vi "McP Position Limit Checker.vi"(1 "Scanning Step":dbl=100.0 min=0.0 format="%.4f", 2 "Old Counter Position":dbl=619.92122 min=0.0 format="%.4f", 3 "New Counter Position":dbl=619.92122 min=0.0 format="%.4f") -> (0 "New Counter Position output":dbl=619.92122 format="%.4f")   [LabVIEW 2025]
doc: "Author: Scott Hannahs <sth@magnet.fsu.edu>\n\nThis software is licensed for use under the “MIT License\"\nCopyright (c) 2025 Scott Hannahs, sth@sth@magnet.sthnet.net\n\nPermission is hereby granted, free of charge, to any person obtaining a copy of this software and associated documentation files (the \"Software\"), to deal in the Software without restriction, including without limitation the rights to use, copy, modify, merge, publish, distribute, sublicense, and/or sell copies of the Software, and to permit persons to whom the Software is furnished to do so, subject to the following conditions: The above copyright notice and this permission notice shall be included in all copies or substantial portions of the Software.\n\nTHE SOFTWARE IS PROVIDED \"AS IS\", WITHOUT WARRANTY OF ANY KIND, EXPRESS OR IMPLIED, INCLUDING BUT NOT LIMITED TO THE WARRANTIES OF MERCHANTABILITY, FITNESS FOR A PARTICULAR PURPOSE AND NONINFRINGEMENT. IN NO EVENT SHALL THE AUTHORS OR COPYRIGHT HOLDERS BE LIABLE FOR ANY CLAIM, DAMAGES OR OTHER LIABILITY, WHETHER IN AN ACTION OF CONTRACT, TORT OR OTHERWISE, ARISING FROM, OUT OF OR IN CONNECTION WITH THE SOFTWARE OR THE USE OR OTHER DEALINGS IN THE SOFTWARE."
panel:
  out "Message":string
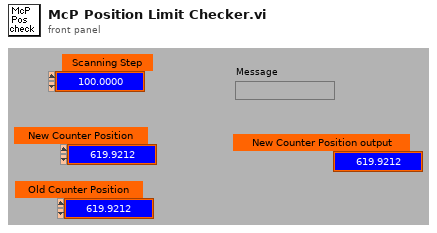
[diagram p1: front panel]
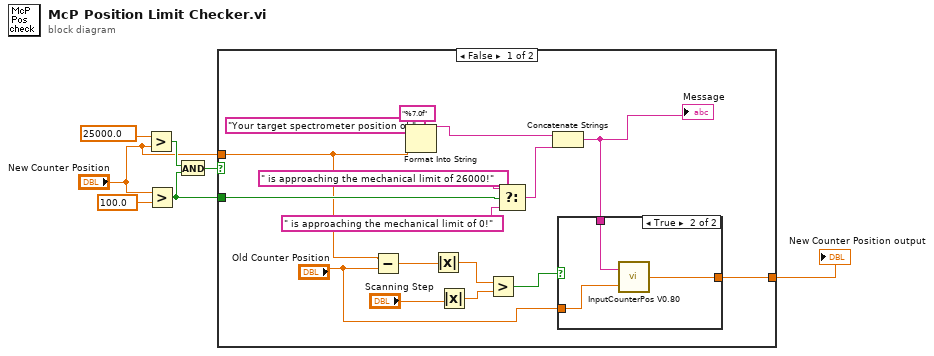
[diagram p0: block diagram]
diagram:
  n1 = Greater?(x=25000.0 ("y"), y="New Counter Position") -> (0:w5:bool)
  n2 = Greater?(x="New Counter Position", y=100.0) -> (0:w2:bool)
  n3 = And(x=w5, y=w2) -> (x .and. y?=w4:bool)
  n4 = case shown="False" w4 {
    tunnel: "New Counter Position" -> [w9 w28]
    tunnel: w2 -> [w17 _]
    tunnel: [w10 w28] -> w1
    frame False {
      n5 = Subtract(x=w9, y="Old Counter Position") -> (x-y=w16:dbl)
      n6 = Format Into String(format string="%7.0f", initial string="Your target spectrometer position of ", w9) -> (resulting string=w21:string)  [unwired: 1 in, 1 out]
      n7 = Absolute Value(x=w16) -> (abs(x)=w14:dbl)
      n8 = Absolute Value(x="Scanning Step") -> (abs(x)=w13:dbl)
      n9 = Greater?(x=w14, y=w13) -> (0:w12:bool)
      n10 = Select(t=" is approaching the mechanical limit of 26000!", s=w17, f=" is approaching the mechanical limit of 0!") -> (s? t:f=w18:string)
      n11 = Concatenate Strings(w21, w18) -> (w11:string)
      "Message" <- w11
      n12 = case shown="True" w12 {
        tunnel: w11 -> [_ w27]
        tunnel: "Old Counter Position" -> [w24 w26]
        tunnel: [w24 w25] -> w10
        frame False {
        }
        frame True {
          n13 = call "InputCounterPos V0.80.vi"("Counter Position"=w26, "Message"=w27) -> ("New Counter Position"=w25:dbl)
        }
      }
    }
    frame True {
    }
  }
  "New Counter Position output" <- w1
